vi "Create String Control.vi"(0 "VI Refnum":refnum<vi>, 2 "Typedef Cluster":refnum<vi>, 5 "Clust Refnum":refnum<vi>, 11 "error in (no error)":errorcluster) -> (4 "Reference String":string, 6 "String ctl ref":refnum<vi>, 15 "error out":errorcluster)   [LabVIEW 2021, in "Converter.lvlib"]
uses:
  Converter.lvlib
  <vilib>/Utility/miscctls.llb/LVPointTypeDef.ctl
  <vilib>/Utility/miscctls.llb/LVPositionTypeDef.ctl
  Converter Reusables/Converter Reusables.lvlib
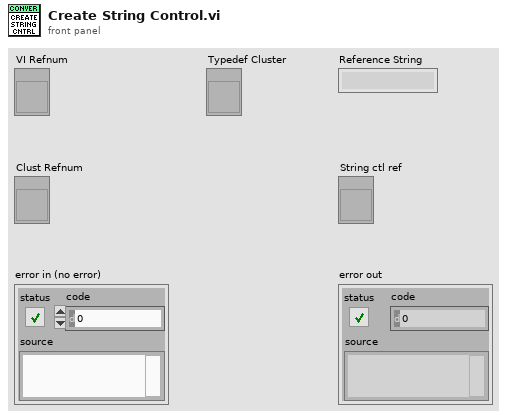
[diagram p1: front panel]
types:
  T1 = typedef "LVPositionTypeDef.ctl" = cluster{"Left":i32, "Top":i32}
  T2 = typedef "LVPointTypeDef.ctl" = cluster{"Horizontal":i16, "Vertical":i16}
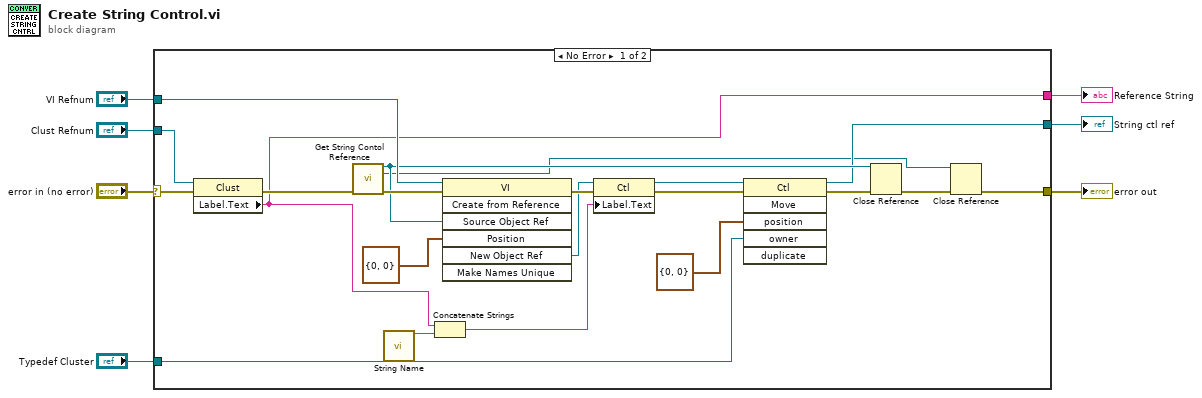
[diagram p0: block diagram]
diagram:
  n1 = case shown="No Error" "error in (no error)" {
    selector: "error in (no error)" -> [w28 w29]
    tunnel: "Clust Refnum" -> [w27 _]
    tunnel: "VI Refnum" -> [w26 _]
    tunnel: [w11 w29] -> w4
    tunnel: [w9 _] -> w3
    tunnel: [w16 _] -> w2
    tunnel: "Typedef Cluster" -> [w14 _]
    frame No Error {
      n2 = property class="Clust"(reference=w27, error in=w28) -> (error out=w25:errorcluster, "Label.Text"=w9:string)  [unwired: 1 out]
      n3 = call "Get String Contol Reference.vi"("error in (no error)"=w25) -> ("String"=w22:refnum<vi>, "vi reference"=w12:refnum<vi>, "error out"=w24:errorcluster)  [unwired: 12 in]
      n4 = call "String Name.vi"() -> ("Postfix"=w8:string)  [unwired: 15 in]
      n5 = Concatenate Strings(w9, w8) -> (w19:string)
      n6 = invoke class="VI" method="Create from Reference"(reference=w26, error in=w24, "Source Object Ref"=w22, "Position"=T2 {"Horizontal"=0, "Vertical"=0}) -> (error out=w21:errorcluster, "New Object Ref"=w20:refnum<vi>)  [unwired: 3 in, 5 out]
      n7 = property class="Ctl"(reference=w20, error in=w21, "Label.Text"=w19) -> (reference out=w18:refnum<vi>, error out=w17:errorcluster)
      n8 = invoke class="Ctl" method="Move"(reference=w18, error in=w17, "position"=T1 {"Left"=0, "Top"=0}, "owner"=w14) -> (reference out=w16:refnum<vi>, error out=w15:errorcluster)  [unwired: 2 in, 4 out]
      n9 = Close Reference(reference=w22, error in (no error)=w15) -> (error out=w10:errorcluster)
      n10 = Close Reference(reference=w12, error in (no error)=w10) -> (error out=w11:errorcluster)
    }
    frame Error {
    }
  }
  "error out" <- w4
  "Reference String" <- w3
  "String ctl ref" <- w2
